vi "Check Instrument Calibration.vi"(7 "Seq Count":i32, 8 "error in (no error)":errorcluster, 11 "Instrument Record":T1) -> (0 "error out":errorcluster, 3 "Cal Expired?":bool)   [LabVIEW 2011]
uses:
  typedefs/Instrument Record.ctl
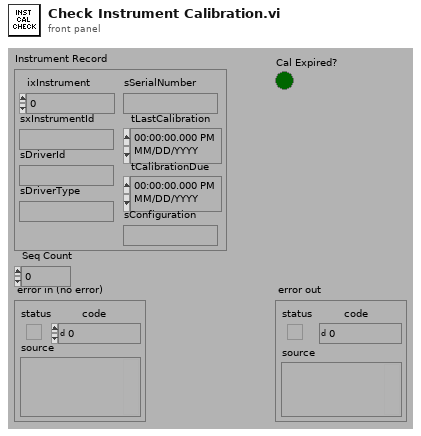
[diagram p1: front panel]
types:
  T1 = typedef "Instrument Record.ctl" = cluster{"ixInstrument":i32, "sxInstrumentId":string, "sDriverId":string, "sDriverType":string, "sSerialNumber":string, "tLastCalibration":timestamp, "tCalibrationDue":timestamp, "sConfiguration":string}
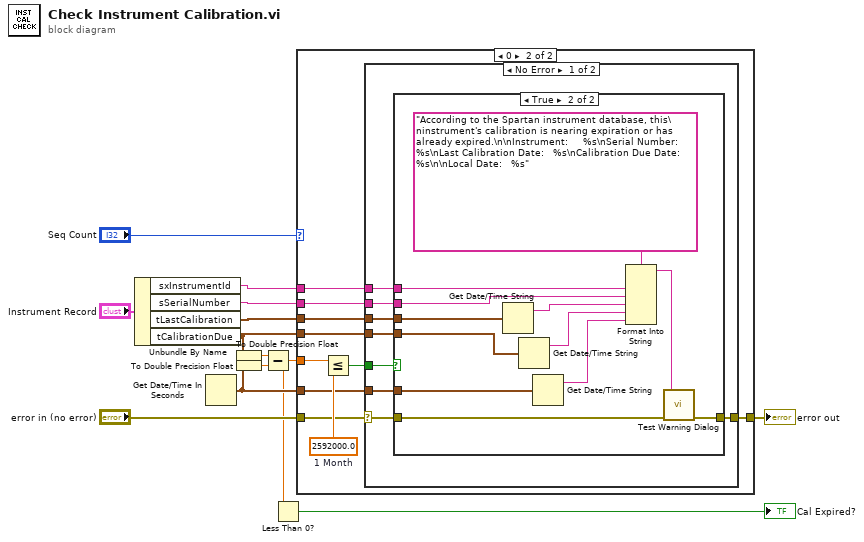
[diagram p0: block diagram]
diagram:
  n1 = Unbundle By Name("Instrument Record") -> ("sxInstrumentId"=w9:string, "sSerialNumber"=w8:string, "tLastCalibration"=w11:timestamp, "tCalibrationDue"=w10:timestamp)
  n2 = Get Date/Time In Seconds() -> (seconds since 1Jan1904=w7:timestamp)
  n3 = To Double Precision Float(number=w10) -> (double precision float=w13:dbl)
  n4 = To Double Precision Float(number=w7) -> (double precision float=w12:dbl)
  n5 = Subtract(x=w13, y=w12) -> (x-y=w3:dbl)
  n6 = Less Than 0?(x=w3) -> (x < 0?=→"Cal Expired?":bool)
  n7 = case shown="0" "Seq Count" {
    tunnel: w11 -> [_ w22]
    tunnel: w10 -> [_ w21]
    tunnel: w9 -> [_ w20]
    tunnel: w8 -> [_ w19]
    tunnel: w7 -> [_ w18]
    tunnel: [w14 w17] -> w5
    tunnel: "error in (no error)" -> [w14 w16]
    tunnel: w3 -> [_ w15]
    frame Default {
      # "Do not run check if it is not the first time the sequence is run."
    }
    frame 0 {
      w24 = 2592000.0  # 1 Month
      n8 = Less Or Equal?(x=w15, y=w24) -> (x <= y?=w23:bool)
      n9 = case shown="No Error" w16 {
        selector: w16 -> [w25 w46]
        tunnel: w23 -> [w32 _]
        tunnel: w22 -> [w31 _]
        tunnel: w21 -> [w30 _]
        tunnel: w20 -> [w29 _]
        tunnel: w19 -> [w28 _]
        tunnel: w18 -> [w27 _]
        tunnel: [w26 w46] -> w17
        frame No Error {
          n10 = case shown="True" w32 {
            tunnel: w25 -> [w33 w45]
            tunnel: [w33 w44] -> w26
            tunnel: w31 -> [_ w39]
            tunnel: w30 -> [_ w37]
            tunnel: w29 -> [_ w41]
            tunnel: w28 -> [_ w40]
            tunnel: w27 -> [_ w35]
            frame False {
            }
            frame True {
              n11 = Get Date/Time String(seconds (now)=w39) -> (date string=w38:string)  [unwired: 3 out]
              n12 = Get Date/Time String(seconds (now)=w37) -> (date string=w36:string)  [unwired: 3 out]
              n13 = Get Date/Time String(seconds (now)=w35) -> (date string=w34:string)  [unwired: 3 out]
              n14 = Format Into String(format string="According to the Spartan instrument database, this\ninstrument's calibration is nearing expiration or has already expired.\n\nInstrument:     %s\nSerial Number:     %s\nLast Calibration Date:   %s\nCalibration Due Date:    %s\n\nLocal Date:   %s", w41, w40, w38, w36, w34) -> (resulting string=w42:string)  [unwired: 2 in, 1 out]
              n15 = call "Test Warning Dialog.vi"("error in (no error)"=w45, "Warning Message"=w42) -> ("error out"=w44:errorcluster)  [unwired: 5 out]
            }
          }
        }
        frame Error {
        }
      }
    }
  }
  "error out" <- w5
